vi "Noti_in.vi"(8 "error in (no error)":errorcluster, 11 "NotifyIcon in":refnum<class "NotifyIcon.lvclass">) -> (0 "error out":errorcluster, 3 "NotifyIcon out":refnum<class "NotifyIcon.lvclass">)   [LabVIEW 2016, in "NotifyIcon.lvclass"]
uses:
  NotifyIcon.lvclass
  NotifyIcon.lvclass/NotifyIcon.ctl
  System.Windows.Forms
  System.Drawing
  ContexMenue/ContexMenue.lvclass
  Icon/Icon.lvclass
  BallonTip/BalloonTip.lvclass
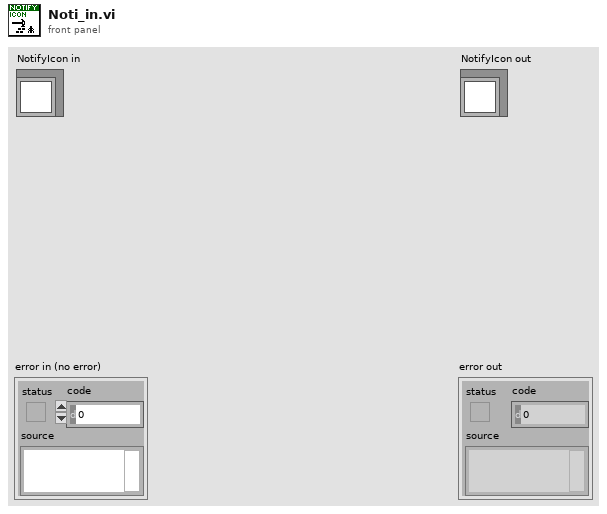
[diagram p1: front panel]
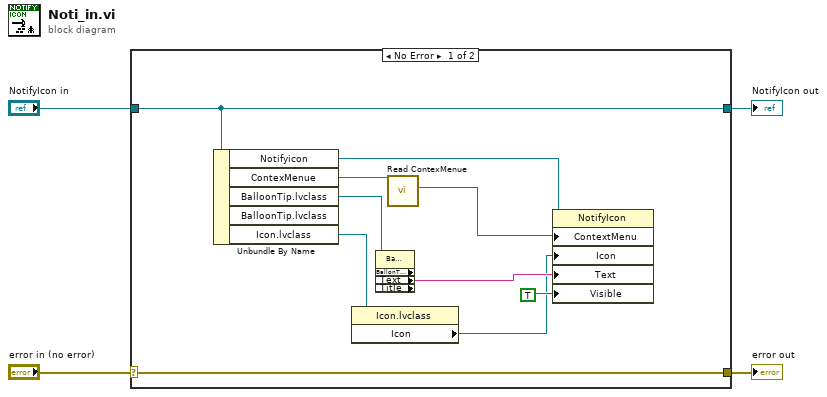
[diagram p0: block diagram]
diagram:
  n1 = case shown="No Error" "error in (no error)" {
    selector: "error in (no error)" -> [w14 w16]
    tunnel: [w14 w16] -> w3
    tunnel: [w13 w15] -> w1
    tunnel: "NotifyIcon in" -> [w13 w15]
    frame No Error {
      n2 = Unbundle By Name(w13) -> ("Notifyicon"=w11:refnum<k24>, "ContexMenue"=w10:refnum<class "ContexMenue.lvclass">, "BalloonTip.lvclass"=w8:refnum<class "BalloonTip.lvclass">, "Icon.lvclass"=w6:refnum<class "Icon.lvclass">)  [unwired: 1 out]
      n3 = property class="Icon.lvclass"(reference=w6) -> ("Icon"=w5:refnum<k24>)  [unwired: 1 in, 2 out]
      n4 = property class="BalloonTip.lvclass" props=["BallonTipText", "Text", "Title"](reference=w8) -> ("Text"=w7:string)  [unwired: 1 in, 4 out]
      n5 = call-dynamic "Read ContexMenue.vi"("ContexMenue in"=w10) -> ("ContexMenue"=w9:refnum<k24>)  [unwired: 8 in, 2 out]
      n6 = property class="NotifyIcon"(reference=w11, "ContextMenu"=w9, "Icon"=w5, "Text"=w7, "Visible"=TRUE) -> ()  [unwired: 1 in, 2 out]
    }
    frame Error {
    }
  }
  "error out" <- w3
  "NotifyIcon out" <- w1
